vi "Connect.vi"(8 "error in (no error)":errorcluster, 9 "Custom Config Data":u8[](array[numeric]) format="%.0x", 10 "Connection Name":string, 11 "RTFIFODouble in":refnum<class "RTFIFODouble.lvclass">) -> (0 "error out":errorcluster, 3 "RTFIFODouble out":refnum<class "RTFIFODouble.lvclass">)   [LabVIEW 2021, in "RTFIFODouble.lvclass"]
uses:
  RTFIFODouble.lvclass
  D:/dev/CIF-LVCore/src/Channels/CIFChannels/CIFChannels.lvclass
  CIFChannels/Typedef/Channel State.ctl
  CIFChannels/CIFChannels.lvclass/CIFChannels.ctl
  RTFIFODouble.lvclass/RTFIFODouble.ctl
  CIFChannels/Accessors/Write Channel State.vi
  CIFChannels/CIFChannels.lvclass
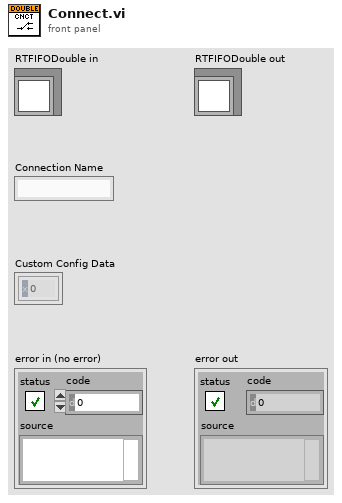
[diagram p1: front panel]
types:
  T1 = typedef "CIFChannels.lvclass/Channel State.ctl" = enum16{"Creating", "Disconnected", "Connecting", "Connected", "Destroyed"}
  T2 = cluster{"read mode":enum16{"polling", "blocking"}, "write mode":enum16{"polling", "blocking"}}
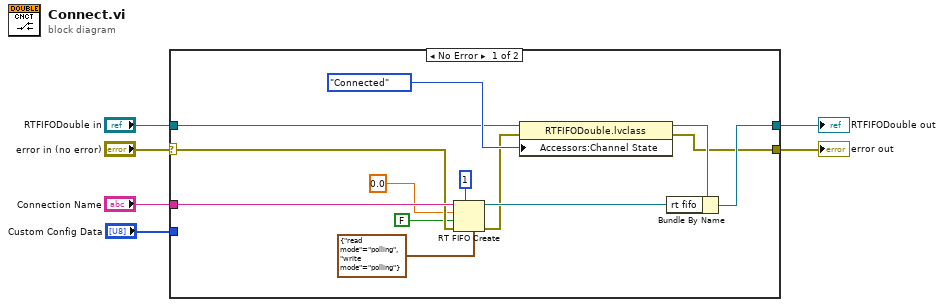
[diagram p0: block diagram]
diagram:
  n1 = case shown="No Error" "error in (no error)" {
    selector: "error in (no error)" -> [w10 w21]
    tunnel: [w11 w21] -> w5
    tunnel: [w15 w20] -> w3
    tunnel: "RTFIFODouble in" -> [w9 w20]
    tunnel: "Connection Name" -> [w19 _]
    tunnel: "Custom Config Data" -> [_ _]
    frame No Error {
      n2 = RT FIFO Create(0:w19, 1:0.0, 2:FALSE ("create if not found? (T)"), 3:w10, 4:u32 1 ("size (10)"), 7:T2 {"read mode"=enum."polling", "write mode"=enum."polling"} ("r/w modes (polling,polling)")) -> (8:w16:refnum<k33>, 11:w12:errorcluster)  [unwired: 2 in, 1 out]
      n3 = property class="RTFIFODouble.lvclass"(reference=w9, error in=w12, "Accessors:Channel State"=Channel_State."Connected" ("Channel State")) -> (reference out=w14:refnum<class "RTFIFODouble.lvclass">, error out=w11:errorcluster)
      n4 = Bundle By Name(cluster=w14, "rt fifo"=w16) -> (w15:refnum<class "RTFIFODouble.lvclass">)
    }
    frame Error {
    }
  }
  "error out" <- w5
  "RTFIFODouble out" <- w3
